vi "2_digit_7_seg_display.vi"() -> ()   [LabVIEW 2019]
panel:
  in  "stop":bool
  out "previous value":u64
  out "increment":u64
  out "e2":bool
  out "f2":bool
  out "c2":bool
  out "b2":bool
  out "d2":bool
  out "g2":bool
  out "a2":bool
  out "e1":bool
  out "f1":bool
  out "c1":bool
  out "b1":bool
  out "d1":bool
  out "g1":bool
  out "a1":bool
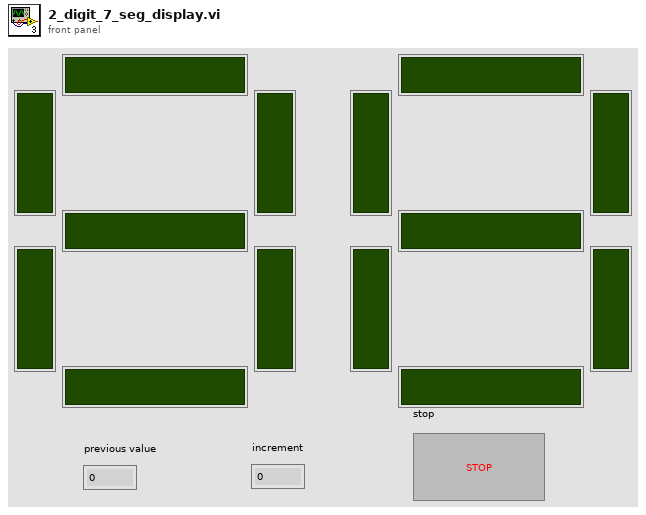
[diagram p1: front panel]
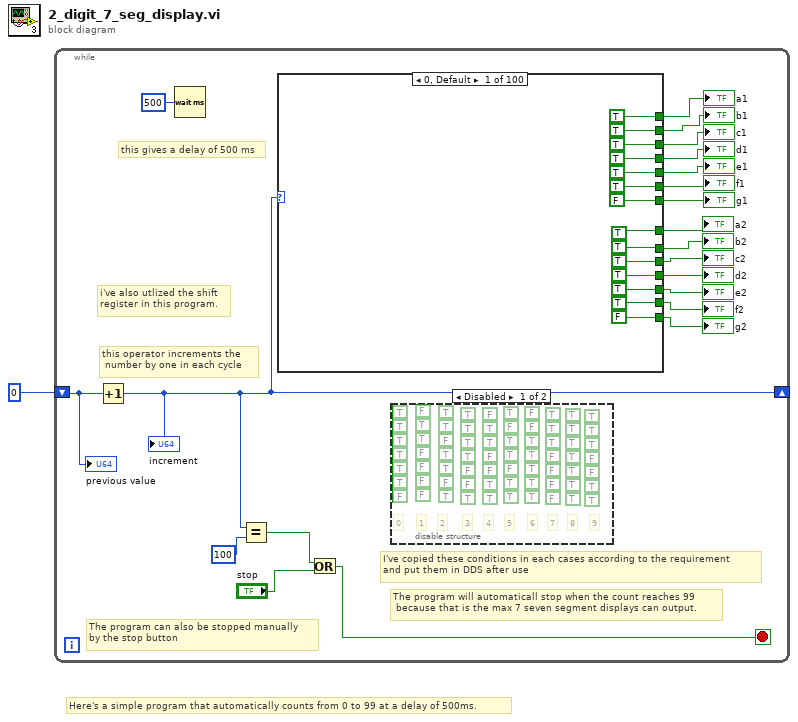
[diagram p0: block diagram]
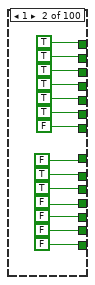
[diagram p3: hidden frame]
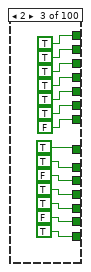
[diagram p4: hidden frame]
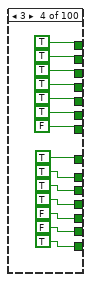
[diagram p5: hidden frame]
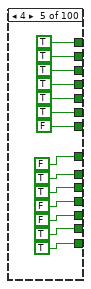
[diagram p6: hidden frame]
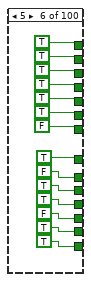
[diagram p7: hidden frame]
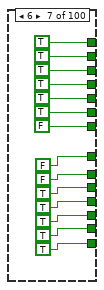
[diagram p8: hidden frame]
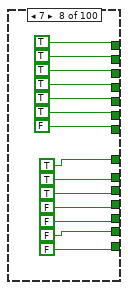
[diagram p9: hidden frame]
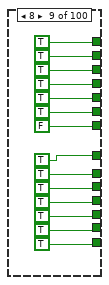
[diagram p10: hidden frame]
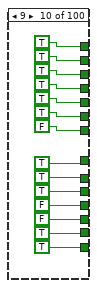
[diagram p11: hidden frame]
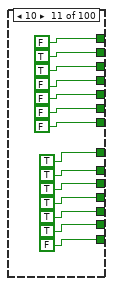
[diagram p12: hidden frame]
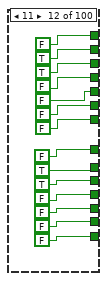
[diagram p13: hidden frame]
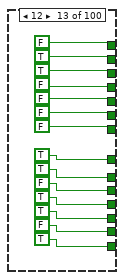
[diagram p14: hidden frame]
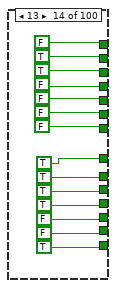
[diagram p15: hidden frame]
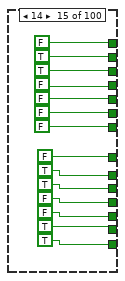
[diagram p16: hidden frame]
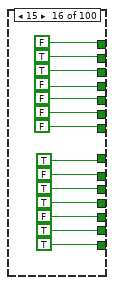
[diagram p17: hidden frame]
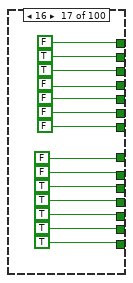
[diagram p18: hidden frame]
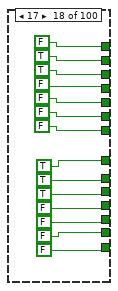
[diagram p19: hidden frame]
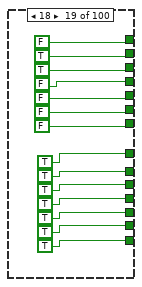
[diagram p20: hidden frame]
diagram:
  # "Here's a simple program that automatically counts from 0 to 99 at a delay of 500ms."
  n1 = while {
    shift-right: [w7] -> _
    shift-left: u64 0 -> [w5]
    stop <- w2 stop-if-true
    # "i've also utlized the shift \nregister in this program."
    # "The program can also be stopped manually\nby the stop button"
    # "this gives a delay of 500 ms"
    # "this operator increments the\n number by one in each cycle"
    # "The program will automaticall stop when the count reaches 99\n because that is the max 7 seven segment displays can output."
    # "I've copied these conditions in each cases according to the requirement\nand put them in DDS after use"
    n2 = Increment(x=w5) -> (x+1=w7:u64)
    "increment" <- w7
    n3 = Wait (ms)(milliseconds to wait=u32 500) -> ()  [unwired: 1 out]
    n4 = Equal?(x=w7, y=u64 100) -> (x = y?=w4:bool)
    n5 = case shown="0, Default" w7 {
      tunnel: [TRUE TRUE TRUE TRUE TRUE TRUE TRUE TRUE TRUE TRUE FALSE FALSE FALSE FALSE FALSE FALSE FALSE FALSE FALSE FALSE TRUE TRUE TRUE TRUE TRUE TRUE TRUE TRUE TRUE TRUE TRUE TRUE TRUE TRUE TRUE TRUE TRUE TRUE TRUE TRUE FALSE FALSE FALSE FALSE FALSE FALSE FALSE FALSE FALSE FALSE TRUE TRUE TRUE TRUE TRUE TRUE TRUE TRUE TRUE TRUE FALSE FALSE FALSE FALSE FALSE FALSE FALSE FALSE FALSE FALSE TRUE TRUE TRUE TRUE TRUE TRUE TRUE TRUE TRUE TRUE TRUE TRUE TRUE TRUE TRUE TRUE TRUE TRUE TRUE TRUE TRUE TRUE TRUE TRUE TRUE TRUE TRUE TRUE TRUE TRUE] -> w22
      tunnel: [TRUE TRUE TRUE TRUE TRUE TRUE TRUE TRUE TRUE TRUE TRUE TRUE TRUE TRUE TRUE TRUE TRUE TRUE TRUE TRUE TRUE TRUE TRUE TRUE TRUE TRUE TRUE TRUE TRUE TRUE TRUE TRUE TRUE TRUE TRUE TRUE TRUE TRUE TRUE TRUE TRUE TRUE TRUE TRUE TRUE TRUE TRUE TRUE TRUE TRUE FALSE FALSE FALSE FALSE FALSE FALSE FALSE FALSE FALSE FALSE FALSE FALSE FALSE FALSE FALSE FALSE FALSE FALSE FALSE FALSE TRUE TRUE TRUE TRUE TRUE TRUE TRUE TRUE TRUE TRUE TRUE TRUE TRUE TRUE TRUE TRUE TRUE TRUE TRUE TRUE TRUE TRUE TRUE TRUE TRUE TRUE TRUE TRUE TRUE TRUE] -> w21
      tunnel: [TRUE TRUE TRUE TRUE TRUE TRUE TRUE TRUE TRUE TRUE TRUE TRUE TRUE TRUE TRUE TRUE TRUE TRUE TRUE TRUE FALSE FALSE FALSE FALSE FALSE FALSE FALSE FALSE FALSE FALSE TRUE TRUE TRUE TRUE TRUE TRUE TRUE TRUE TRUE TRUE TRUE TRUE TRUE TRUE TRUE TRUE TRUE TRUE TRUE TRUE TRUE TRUE TRUE TRUE TRUE TRUE TRUE TRUE TRUE TRUE TRUE TRUE TRUE TRUE TRUE TRUE TRUE TRUE TRUE TRUE TRUE TRUE TRUE TRUE TRUE TRUE TRUE TRUE TRUE TRUE TRUE TRUE TRUE TRUE TRUE TRUE TRUE TRUE TRUE TRUE TRUE TRUE TRUE TRUE TRUE TRUE TRUE TRUE TRUE TRUE] -> w20
      tunnel: [TRUE TRUE TRUE TRUE TRUE TRUE TRUE TRUE TRUE TRUE FALSE FALSE FALSE FALSE FALSE FALSE FALSE FALSE FALSE FALSE TRUE TRUE TRUE TRUE TRUE TRUE TRUE TRUE TRUE TRUE TRUE TRUE TRUE TRUE TRUE TRUE TRUE TRUE TRUE TRUE FALSE FALSE FALSE FALSE FALSE FALSE FALSE FALSE FALSE FALSE TRUE TRUE TRUE TRUE TRUE TRUE TRUE TRUE TRUE TRUE TRUE TRUE TRUE TRUE TRUE TRUE TRUE TRUE TRUE TRUE FALSE FALSE FALSE FALSE FALSE FALSE FALSE FALSE FALSE FALSE TRUE TRUE TRUE TRUE TRUE TRUE TRUE TRUE TRUE TRUE FALSE FALSE FALSE FALSE FALSE FALSE FALSE FALSE FALSE FALSE] -> w19
      tunnel: [TRUE TRUE TRUE TRUE TRUE TRUE TRUE TRUE TRUE TRUE FALSE FALSE FALSE FALSE FALSE FALSE FALSE FALSE FALSE FALSE TRUE TRUE TRUE TRUE TRUE TRUE TRUE TRUE TRUE TRUE FALSE FALSE FALSE FALSE FALSE FALSE FALSE FALSE FALSE FALSE FALSE FALSE FALSE FALSE FALSE FALSE FALSE FALSE FALSE FALSE FALSE FALSE FALSE FALSE FALSE FALSE FALSE FALSE FALSE FALSE TRUE TRUE TRUE TRUE TRUE TRUE TRUE TRUE TRUE TRUE FALSE FALSE FALSE FALSE FALSE FALSE FALSE FALSE FALSE FALSE TRUE TRUE TRUE TRUE TRUE TRUE TRUE TRUE TRUE TRUE FALSE FALSE FALSE FALSE FALSE FALSE FALSE FALSE FALSE FALSE] -> w18
      tunnel: [TRUE TRUE TRUE TRUE TRUE TRUE TRUE TRUE TRUE TRUE FALSE FALSE FALSE FALSE FALSE FALSE FALSE FALSE FALSE FALSE FALSE FALSE FALSE FALSE FALSE FALSE FALSE FALSE FALSE FALSE FALSE FALSE FALSE FALSE FALSE FALSE FALSE FALSE FALSE FALSE TRUE TRUE TRUE TRUE TRUE TRUE TRUE TRUE TRUE TRUE TRUE TRUE TRUE TRUE TRUE TRUE TRUE TRUE TRUE TRUE TRUE TRUE TRUE TRUE TRUE TRUE TRUE TRUE TRUE TRUE FALSE FALSE FALSE FALSE FALSE FALSE FALSE FALSE FALSE FALSE TRUE TRUE TRUE TRUE TRUE TRUE TRUE TRUE TRUE TRUE TRUE TRUE TRUE TRUE TRUE TRUE TRUE TRUE TRUE TRUE] -> w17
      tunnel: [FALSE FALSE FALSE FALSE FALSE FALSE FALSE FALSE FALSE FALSE FALSE FALSE FALSE FALSE FALSE FALSE FALSE FALSE FALSE FALSE TRUE TRUE TRUE TRUE TRUE TRUE TRUE TRUE TRUE TRUE TRUE TRUE TRUE TRUE TRUE TRUE TRUE TRUE TRUE TRUE TRUE TRUE TRUE TRUE TRUE TRUE TRUE TRUE TRUE TRUE TRUE TRUE TRUE TRUE TRUE TRUE TRUE TRUE TRUE TRUE TRUE TRUE TRUE TRUE TRUE TRUE TRUE TRUE TRUE TRUE FALSE FALSE FALSE FALSE FALSE FALSE FALSE FALSE FALSE FALSE TRUE TRUE TRUE TRUE TRUE TRUE TRUE TRUE TRUE TRUE TRUE TRUE TRUE TRUE TRUE TRUE TRUE TRUE TRUE TRUE] -> w16
      tunnel: [TRUE FALSE TRUE TRUE FALSE TRUE FALSE TRUE TRUE TRUE TRUE FALSE TRUE TRUE FALSE TRUE FALSE TRUE TRUE TRUE TRUE FALSE TRUE TRUE FALSE TRUE FALSE TRUE TRUE TRUE TRUE FALSE TRUE TRUE FALSE TRUE FALSE TRUE TRUE TRUE TRUE FALSE TRUE TRUE FALSE TRUE FALSE TRUE TRUE TRUE TRUE FALSE TRUE TRUE FALSE TRUE FALSE TRUE TRUE TRUE TRUE FALSE TRUE TRUE FALSE TRUE FALSE TRUE TRUE TRUE TRUE FALSE TRUE TRUE FALSE TRUE FALSE TRUE TRUE TRUE TRUE FALSE TRUE TRUE FALSE TRUE FALSE TRUE TRUE TRUE TRUE FALSE TRUE TRUE FALSE TRUE FALSE TRUE TRUE TRUE] -> w15
      tunnel: [TRUE TRUE TRUE TRUE TRUE FALSE FALSE TRUE TRUE TRUE TRUE TRUE TRUE TRUE TRUE FALSE FALSE TRUE TRUE TRUE TRUE TRUE TRUE TRUE TRUE FALSE FALSE TRUE TRUE TRUE TRUE TRUE TRUE TRUE TRUE FALSE FALSE TRUE TRUE TRUE TRUE TRUE TRUE TRUE TRUE FALSE FALSE TRUE TRUE TRUE TRUE TRUE TRUE TRUE TRUE FALSE FALSE TRUE TRUE TRUE TRUE TRUE TRUE TRUE TRUE FALSE FALSE TRUE TRUE TRUE TRUE TRUE TRUE TRUE TRUE FALSE FALSE TRUE TRUE TRUE TRUE TRUE TRUE TRUE TRUE FALSE FALSE TRUE TRUE TRUE TRUE TRUE TRUE TRUE TRUE FALSE FALSE TRUE TRUE TRUE] -> w14
      tunnel: [TRUE TRUE FALSE TRUE TRUE TRUE TRUE TRUE TRUE TRUE TRUE TRUE FALSE TRUE TRUE TRUE TRUE TRUE TRUE TRUE TRUE TRUE FALSE TRUE TRUE TRUE TRUE TRUE TRUE TRUE TRUE TRUE FALSE TRUE TRUE TRUE TRUE TRUE TRUE TRUE TRUE TRUE FALSE TRUE TRUE TRUE TRUE TRUE TRUE TRUE TRUE TRUE FALSE TRUE TRUE TRUE TRUE TRUE TRUE TRUE TRUE TRUE FALSE TRUE TRUE TRUE TRUE TRUE TRUE TRUE TRUE TRUE FALSE TRUE TRUE TRUE TRUE TRUE TRUE TRUE TRUE TRUE FALSE TRUE TRUE TRUE TRUE TRUE TRUE TRUE TRUE TRUE FALSE TRUE TRUE TRUE TRUE TRUE TRUE TRUE] -> w13
      tunnel: [TRUE FALSE TRUE TRUE FALSE TRUE TRUE FALSE TRUE FALSE TRUE FALSE TRUE TRUE FALSE TRUE TRUE FALSE TRUE FALSE TRUE FALSE TRUE TRUE FALSE TRUE TRUE FALSE TRUE FALSE TRUE FALSE TRUE TRUE FALSE TRUE TRUE FALSE TRUE FALSE TRUE FALSE TRUE TRUE FALSE TRUE TRUE FALSE TRUE FALSE TRUE FALSE TRUE TRUE FALSE TRUE TRUE FALSE TRUE FALSE TRUE FALSE TRUE TRUE FALSE TRUE TRUE FALSE TRUE FALSE TRUE FALSE TRUE TRUE FALSE TRUE TRUE FALSE TRUE FALSE TRUE FALSE TRUE TRUE FALSE TRUE TRUE FALSE TRUE FALSE TRUE FALSE TRUE TRUE FALSE TRUE TRUE FALSE TRUE FALSE] -> w12
      tunnel: [TRUE FALSE TRUE FALSE FALSE FALSE TRUE FALSE TRUE FALSE TRUE FALSE TRUE FALSE FALSE FALSE TRUE FALSE TRUE FALSE TRUE FALSE TRUE FALSE FALSE FALSE TRUE FALSE TRUE FALSE TRUE FALSE TRUE FALSE FALSE FALSE TRUE FALSE TRUE FALSE TRUE FALSE TRUE FALSE FALSE FALSE TRUE FALSE TRUE FALSE TRUE FALSE TRUE FALSE FALSE FALSE TRUE FALSE TRUE FALSE TRUE FALSE TRUE FALSE FALSE FALSE TRUE FALSE TRUE FALSE TRUE FALSE TRUE FALSE FALSE FALSE TRUE FALSE TRUE FALSE TRUE FALSE TRUE FALSE FALSE FALSE TRUE FALSE TRUE FALSE TRUE FALSE TRUE FALSE FALSE FALSE TRUE FALSE TRUE FALSE] -> w11
      tunnel: [TRUE FALSE FALSE FALSE TRUE TRUE TRUE FALSE TRUE TRUE TRUE FALSE FALSE FALSE TRUE TRUE TRUE FALSE TRUE TRUE TRUE FALSE FALSE FALSE TRUE TRUE TRUE FALSE TRUE TRUE TRUE FALSE FALSE FALSE TRUE TRUE TRUE FALSE TRUE TRUE TRUE FALSE FALSE FALSE TRUE TRUE TRUE FALSE TRUE TRUE TRUE FALSE FALSE FALSE TRUE TRUE TRUE FALSE TRUE TRUE TRUE FALSE FALSE FALSE TRUE TRUE TRUE FALSE TRUE TRUE TRUE FALSE FALSE FALSE TRUE TRUE TRUE FALSE TRUE TRUE TRUE FALSE FALSE FALSE TRUE TRUE TRUE FALSE TRUE TRUE TRUE FALSE FALSE FALSE TRUE TRUE TRUE FALSE TRUE TRUE] -> w10
      tunnel: [FALSE FALSE TRUE TRUE TRUE TRUE TRUE FALSE TRUE TRUE FALSE FALSE TRUE TRUE TRUE TRUE TRUE FALSE TRUE TRUE FALSE FALSE TRUE TRUE TRUE TRUE TRUE FALSE TRUE TRUE FALSE FALSE TRUE TRUE TRUE TRUE TRUE FALSE TRUE TRUE FALSE FALSE TRUE TRUE TRUE TRUE TRUE FALSE TRUE TRUE FALSE FALSE TRUE TRUE TRUE TRUE TRUE FALSE TRUE TRUE FALSE FALSE TRUE TRUE TRUE TRUE TRUE FALSE TRUE TRUE FALSE FALSE TRUE TRUE TRUE TRUE TRUE FALSE TRUE TRUE FALSE FALSE TRUE TRUE TRUE TRUE TRUE FALSE TRUE TRUE FALSE FALSE TRUE TRUE TRUE TRUE TRUE FALSE TRUE TRUE] -> w9
      frame 0, Default {
      }
      frame 1 {
        (unwired) FALSE
      }
      frame 2 {
      }
      frame 3 {
      }
      frame 4 {
      }
      frame 5 {
      }
      frame 6 {
      }
      frame 7 {
      }
      frame 8 {
      }
      frame 9 {
      }
      frame 10 {
        (unwired) FALSE
      }
      frame 11 {
        (unwired) FALSE
        (unwired) FALSE
      }
      frame 12 {
        (unwired) FALSE
      }
      frame 13 {
        (unwired) FALSE
      }
      frame 14 {
        (unwired) FALSE
      }
      frame 15 {
        (unwired) FALSE
      }
      frame 16 {
        (unwired) FALSE
      }
      frame 17 {
        (unwired) FALSE
      }
      frame 18 {
        (unwired) FALSE
      }
      frame 19 {
        (unwired) FALSE
      }
      frame 20 {
      }
      frame 21 {
        (unwired) FALSE
      }
      frame 22 {
      }
      frame 23 {
      }
      frame 24 {
      }
      frame 25 {
      }
      frame 26 {
      }
      frame 27 {
      }
      frame 28 {
      }
      frame 29 {
      }
      frame 30 {
      }
      frame 31 {
        (unwired) FALSE
      }
      frame 32 {
      }
      frame 33 {
      }
      frame 34 {
      }
      frame 35 {
      }
      frame 36 {
      }
      frame 37 {
      }
      frame 38 {
      }
      frame 39 {
      }
      frame 40 {
      }
      frame 41 {
        (unwired) FALSE
      }
      frame 42 {
      }
      frame 43 {
      }
      frame 44 {
      }
      frame 45 {
      }
      frame 46 {
      }
      frame 47 {
      }
      frame 48 {
      }
      frame 49 {
      }
      frame 50 {
      }
      frame 51 {
        (unwired) FALSE
      }
      frame 52 {
      }
      frame 53 {
      }
      frame 54 {
      }
      frame 55 {
      }
      frame 56 {
      }
      frame 57 {
      }
      frame 58 {
      }
      frame 59 {
      }
      frame 60 {
      }
      frame 61 {
        (unwired) FALSE
      }
      frame 62 {
      }
      frame 63 {
      }
      frame 64 {
      }
      frame 65 {
      }
      frame 66 {
      }
      frame 67 {
      }
      frame 68 {
      }
      frame 69 {
      }
      frame 70 {
      }
      frame 71 {
        (unwired) FALSE
      }
      frame 72 {
      }
      frame 73 {
      }
      frame 74 {
      }
      frame 75 {
      }
      frame 76 {
      }
      frame 77 {
      }
      frame 78 {
      }
      frame 79 {
      }
      frame 80 {
      }
      frame 81 {
        (unwired) FALSE
      }
      frame 82 {
      }
      frame 83 {
      }
      frame 84 {
      }
      frame 85 {
      }
      frame 86 {
      }
      frame 87 {
      }
      frame 88 {
      }
      frame 89 {
      }
      frame 90 {
      }
      frame 91 {
        (unwired) FALSE
      }
      frame 92 {
      }
      frame 93 {
      }
      frame 94 {
      }
      frame 95 {
      }
      frame 96 {
      }
      frame 97 {
      }
      frame 98 {
      }
      frame 99 {
      }
    }
    "a1" <- w22
    "g1" <- w16
    "d1" <- w19
    "b1" <- w21
    "c1" <- w20
    "f1" <- w17
    "e1" <- w18
    "a2" <- w15
    "g2" <- w9
    "d2" <- w12
    "b2" <- w14
    "c2" <- w13
    "f2" <- w10
    "e2" <- w11
    n6 = Or(x=w4, y="stop") -> (x .or. y?=w2:bool)
    n7 = disable-structure shown="Disabled" {
      frame Disabled {
        (unwired) TRUE
        (unwired) FALSE
        (unwired) TRUE
        (unwired) TRUE
        (unwired) FALSE
        (unwired) TRUE
        (unwired) TRUE
        (unwired) FALSE
        (unwired) TRUE
        (unwired) TRUE
        (unwired) FALSE
        (unwired) FALSE
        (unwired) TRUE
        (unwired) TRUE
        (unwired) TRUE
        (unwired) TRUE
        (unwired) TRUE
        (unwired) TRUE
        (unwired) TRUE
        (unwired) TRUE
        (unwired) TRUE
        (unwired) TRUE
        (unwired) FALSE
        (unwired) FALSE
        (unwired) FALSE
        (unwired) FALSE
        (unwired) TRUE
        (unwired) TRUE
        (unwired) TRUE
        (unwired) TRUE
        (unwired) TRUE
        (unwired) TRUE
        (unwired) TRUE
        (unwired) TRUE
        (unwired) FALSE
        (unwired) FALSE
        (unwired) TRUE
        (unwired) TRUE
        (unwired) FALSE
        (unwired) TRUE
        (unwired) TRUE
        (unwired) FALSE
        (unwired) TRUE
        (unwired) TRUE
        (unwired) TRUE
        (unwired) FALSE
        (unwired) FALSE
        (unwired) TRUE
        (unwired) TRUE
        (unwired) FALSE
        (unwired) TRUE
        (unwired) FALSE
        (unwired) FALSE
        (unwired) TRUE
        (unwired) TRUE
        (unwired) TRUE
        (unwired) TRUE
        (unwired) FALSE
        (unwired) FALSE
        (unwired) FALSE
        (unwired) FALSE
        (unwired) TRUE
        (unwired) TRUE
        (unwired) FALSE
        (unwired) FALSE
        (unwired) TRUE
        (unwired) TRUE
        (unwired) TRUE
        (unwired) TRUE
        (unwired) TRUE
        (unwired) TRUE
        # "9"
        # "8"
        # "7"
        # "6"
        # "5"
        # "4"
        # "3"
        # "2"
        # "1"
        # "0"
      }
      frame Enabled {
      }
    }
    "previous value" <- w5
  }
